vi "测试demo.vi"() -> ()   [LabVIEW 2014]
panel:
  out "Image":T1(plugin-control)
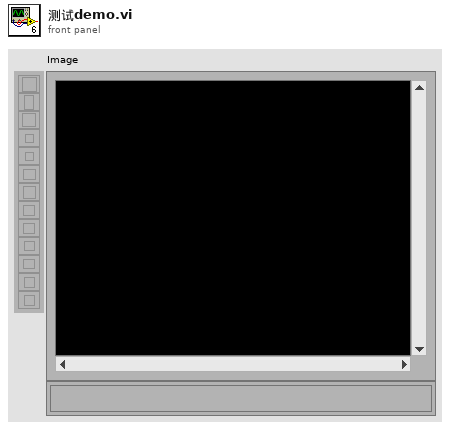
[diagram p1: front panel]
types:
  T1 = typedef "IMAQ Image.ctl" = refnum<image>
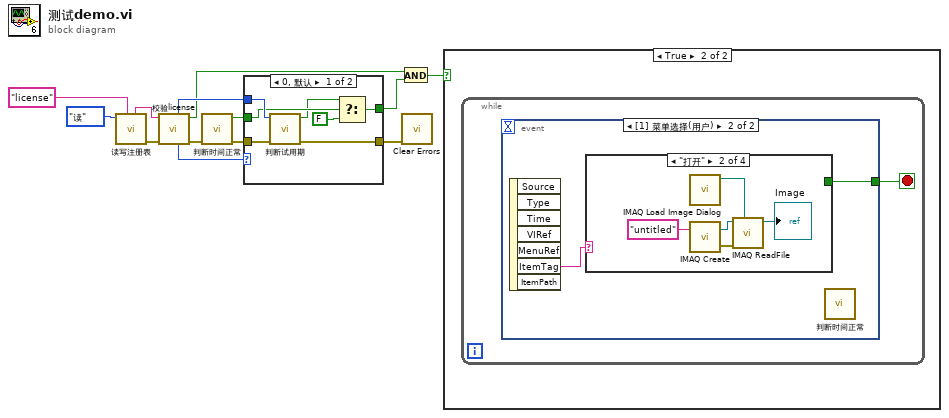
[diagram p0: block diagram]
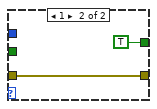
[diagram p2: hidden frame]
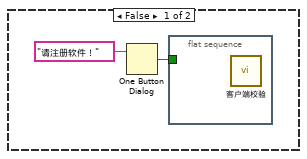
[diagram p3: hidden frame]
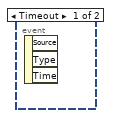
[diagram p4: hidden frame]
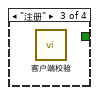
[diagram p6: hidden frame]
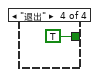
[diagram p7: hidden frame]
diagram:
  n1 = call "读写注册表.vi"("键名称"="license", "读/写"=enum16{"读", "写"}."读") -> ("error out"=w13:errorcluster, "键内容"=w10:string)  [unwired: 8 in]
  n2 = call "校验license.vi"("error in (no error)"=w13, "license"=w10) -> ("error out"=w9:errorcluster, "license正确"=w4:bool, "授权类型"=w8:i32, "T"=w7:u32)  [unwired: 6 in]
  n3 = call "判断时间正常.vi"("error in (no error)"=w9) -> ("error out"=w6:errorcluster, "时间正常"=w3:bool)  [unwired: 9 in]
  n4 = case shown="0, 默认" w8 {
    tunnel: w7 -> [w20 _]
    tunnel: [w15 TRUE ("试用期内")] -> w5
    tunnel: w6 -> [w19 w21]
    tunnel: w3 -> [w18 _]
    tunnel: [w14 w21] -> w1
    frame 0, Default {
      n5 = call "判断试用期.vi"("error in (no error)"=w19, "T"=w20) -> ("error out"=w14:errorcluster, "试用期内"=w17:bool)  [unwired: 8 in]
      n6 = Select(t=w17, s=w18, f=FALSE) -> (s? t:f=w15:bool)
    }
    frame 1 {
    }
  }
  n7 = And(x=w4, y=w5) -> (x .and. y?=w2:bool)
  n8 = call <vilib>:"Clear Errors.vi"("error in (no error)"=w1) -> ()  [unwired: 5 in, 2 out]
  n9 = case shown="True" w2 {
    frame False {
      n10 = One Button Dialog(message="请注册软件！" ("消息")) -> (true=w23:bool)  [unwired: 1 in]
      n11 = flat-sequence {
        tunnel: w23 -> [_]
        frame #0 {
          n12 = call "客户端校验.vi"() -> ()  [unwired: 12 in]
        }
      }
    }
    frame True {
      n13 = while {
        stop <- w25 stop-if-true
        n14 = event shown="[1] 菜单选择(用户)" {
          selector: _ -> [_ _]
          dyn-events: _ -> [_ _]
          timeout: _ -> [_ _]
          tunnel: [_ w26] -> w25
          event Timeout {
            n15 = event-data() -> ()  [unwired: 1 in, 3 out]
          }
          event Menu Selection (User) {
            n16 = event-data() -> ("ItemTag"=w27:string)  [unwired: 1 in, 6 out]
            n17 = case shown="\"打开\"" w27 {
              tunnel: [_ _ _ TRUE] -> w26
              frame "假", Default {
              }
              frame "打开" {
                n18 = call "IMAQ Load Image Dialog"() -> ("Path"=w32:path)  [unwired: 9 in, 2 out]
                n19 = call "IMAQ Create"("Image Name"="untitled") -> ("New Image"=w30:T1, "error out"=w29:errorcluster)  [unwired: 4 in]
                n20 = call "IMAQ ReadFile"("File Path"=w32, "error in (no error)"=w29, "Image"=w30) -> ("Image Out"=→"Image":T1)  [unwired: 4 in, 4 out]
              }
              frame "注册" {
                n21 = call "客户端校验.vi"() -> ()  [unwired: 12 in]
              }
              frame "退出" {
              }
            }
            n22 = call "判断时间正常.vi"() -> ()  [unwired: 10 in, 2 out]
          }
        }
      }
    }
  }
